vi "lf-condition-1122.vi"() -> ()   [LabVIEW 2019]
panel:
  out "Navigate Tree:Get Parent":string
  out "数字":i32
  in  "sce-pannel":T1 {"pannel"."ID" format="%02x"}
  out "节点列表":T2(array[cluster])
  in  "Action":string(combo) caption="动作"
  in  "节点-操作 9":T3={"ID"=0, "type"="dev", "flag"="", "name"="", "Act"={"Attribute"="dev", "Action"="", "Value"=0.0}} caption="簇 7" {"ID" format="%02x"}
  out "节点引用数组":refnum<vi>[](array[refnum])
  in  "节点-操作 4":T3={"ID"=0, "type"="dev", "flag"="", "name"="", "Act"={"Attribute"="dev", "Action"="", "Value"=0.0}} caption="簇 7" {"ID" format="%02x"}
  in  "节点-操作 3":T3={"ID"=0, "type"="dev", "flag"="", "name"="", "Act"={"Attribute"="dev", "Action"="", "Value"=0.0}} caption="簇 7" {"ID" format="%02x"}
  in  "节点-操作 2":T3={"ID"=0, "type"="dev", "flag"="", "name"="", "Act"={"Attribute"="dev", "Action"="", "Value"=0.0}} caption="簇 7" {"ID" format="%02x"}
  in  "节点-操作":T3={"ID"=0, "type"="dev", "flag"="", "name"="", "Act"={"Attribute"="dev", "Action"="", "Value"=0.0}} caption="簇 7" {"ID" format="%02x"}
  in  "模式列表":T4(array[cluster]) {"sce-pannel-list"."pannel"."ID" format="%02x"}
  in  "节点-操作 5":T3={"ID"=0, "type"="dev", "flag"="", "name"="", "Act"={"Attribute"="dev", "Action"="", "Value"=0.0}} caption="簇 7" {"ID" format="%02x"}
  in  "选项卡控件":enum32{"选项卡 1", "选项卡 2"}(tab)
  in  "面板地址 2":u8 format="%02d"
  in  "添加面板":bool
  in  "单选按钮 2":T5(radio)
  in  "簇 6":T6={"ID"=0, "Attribute"="dev", "Action"="", "name"=""} {"ID" format="%02x"}
  in  "簇 5":T6={"ID"=0, "Attribute"="dev", "Action"="", "name"=""} {"ID" format="%02x"}
  in  "簇 4":T6={"ID"=0, "Attribute"="dev", "Action"="", "name"=""} {"ID" format="%02x"}
  in  "簇 3":T6={"ID"=0, "Attribute"="dev", "Action"="", "name"=""} {"ID" format="%02x"}
  in  "簇 2":T6={"ID"=0, "Attribute"="dev", "Action"="", "name"=""} {"ID" format="%02.0f"}
  in  "簇 1":T6={"ID"=0, "Attribute"="dev", "Action"="", "name"=""} {"ID" format="%02x"}
  in  "节点-操作 26":T3={"ID"=0, "type"="dev", "flag"="", "name"="", "Act"={"Attribute"="dev", "Action"="", "Value"=0.0}} caption="簇 7" {"ID" format="%02x"}
  in  "节点-操作 23":T3={"ID"=0, "type"="dev", "flag"="", "name"="", "Act"={"Attribute"="dev", "Action"="", "Value"=0.0}} caption="簇 7" {"ID" format="%02x"}
  in  "节点-操作 25":T3={"ID"=0, "type"="dev", "flag"="", "name"="", "Act"={"Attribute"="dev", "Action"="", "Value"=0.0}} caption="簇 7" {"ID" format="%02x"}
  in  "节点-操作 24":T3={"ID"=0, "type"="dev", "flag"="", "name"="", "Act"={"Attribute"="dev", "Action"="", "Value"=0.0}} caption="簇 7" {"ID" format="%02x"}
  in  "节点-操作 22":T3={"ID"=0, "type"="dev", "flag"="", "name"="", "Act"={"Attribute"="dev", "Action"="", "Value"=0.0}} caption="簇 7" {"ID" format="%02x"}
  in  "节点-操作 21":T3={"ID"=0, "type"="dev", "flag"="", "name"="", "Act"={"Attribute"="dev", "Action"="", "Value"=0.0}} caption="簇 7" {"ID" format="%02x"}
  in  "面板地址":string(combo)
  in  "模式":string(combo)
  in  "添加设备":bool
  in  "节点-输出":T7(array[cluster])
  in  "场景":string(tree)
  out "node":T7(array[cluster])
  in  "停止":bool
  out "pannel-id-list":string[](array[string])
  out "Node-list":T8(array[cluster])
  in  "Node-model":T9
  in  "pannel-list":T10(array[cluster])
  in  "panel":string(tree)
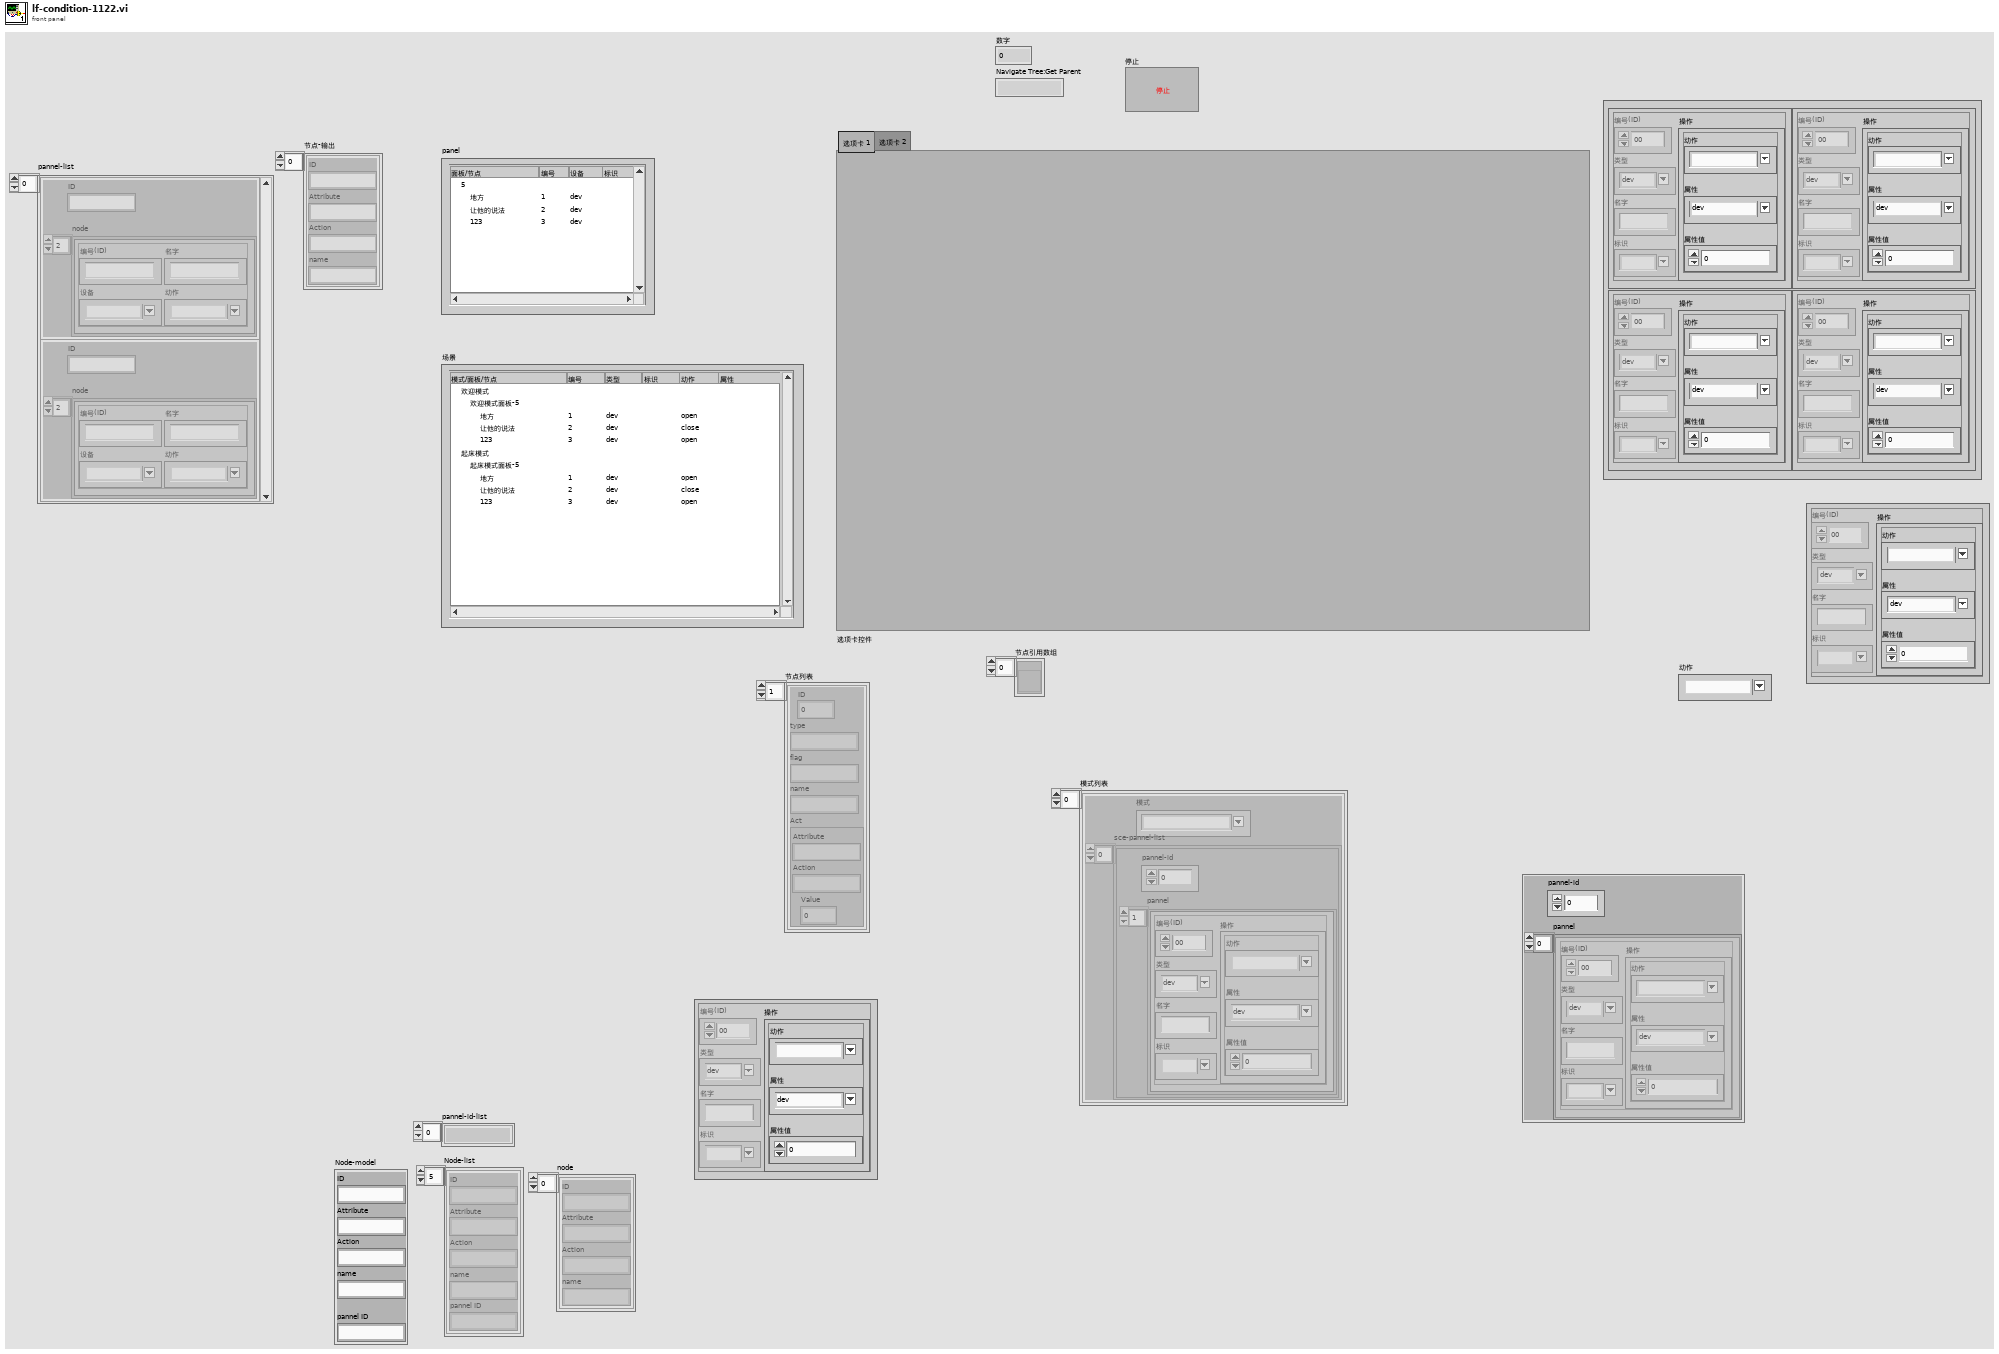
[diagram p1: front panel]
types:
  T1 = cluster{"pannel":cluster{"ID":u8, "type":string, "flag":string, "name":string, "Act":cluster{"Attribute":string, "Action":string, "Value":dbl}}[], "pannel-id":dbl}
  T2 = cluster{"ID":u8, "type":string, "flag":string, "name":string, "Act":cluster{"Attribute":string, "Action":string, "Value":dbl}}[]
  T3 = cluster{"ID":u8, "type":string, "flag":string, "name":string, "Act":cluster{"Attribute":string, "Action":string, "Value":dbl}}
  T4 = cluster{"模式":string, "sce-pannel-list":cluster{"pannel":cluster{"ID":u8, "type":string, "flag":string, "name":string, "Act":cluster{"Attribute":string, "Action":string, "Value":dbl}}[], "pannel-id":dbl}[]}[]
  T5 = enum32{"单键面板", "双键面板", "三键面板", "四键面板", "六键面板", "调光面板"}
  T6 = cluster{"ID":u8, "Attribute":string, "Action":string, "name":string}
  T7 = cluster{"ID":string, "Attribute":string, "Action":string, "name":string}[]
  T8 = cluster{"ID":string, "Attribute":string, "Action":string, "name":string, "pannel ID":string}[]
  T9 = cluster{"ID":string, "Attribute":string, "Action":string, "name":string, "pannel ID":string}
  T10 = cluster{"node":cluster{"ID":string, "Attribute":string, "Action":string, "name":string}[], "ID":string}[]
  T11 = cluster{"node":cluster{"ID":string, "Attribute":string, "Action":string, "name":string}[], "ID":string}
  T12 = enum8{"Enabled", "Disabled", "Disabled and Grayed Out"}
  T13 = cluster{"模式":string, "sce-pannel-list":cluster{"pannel":cluster{"ID":u8, "type":string, "flag":string, "name":string, "Act":cluster{"Attribute":string, "Action":string, "Value":dbl}}[], "pannel-id":dbl}[]}
  T14 = cluster{"ID":u8, "Attribute":string, "Action":string, "name":string}[]
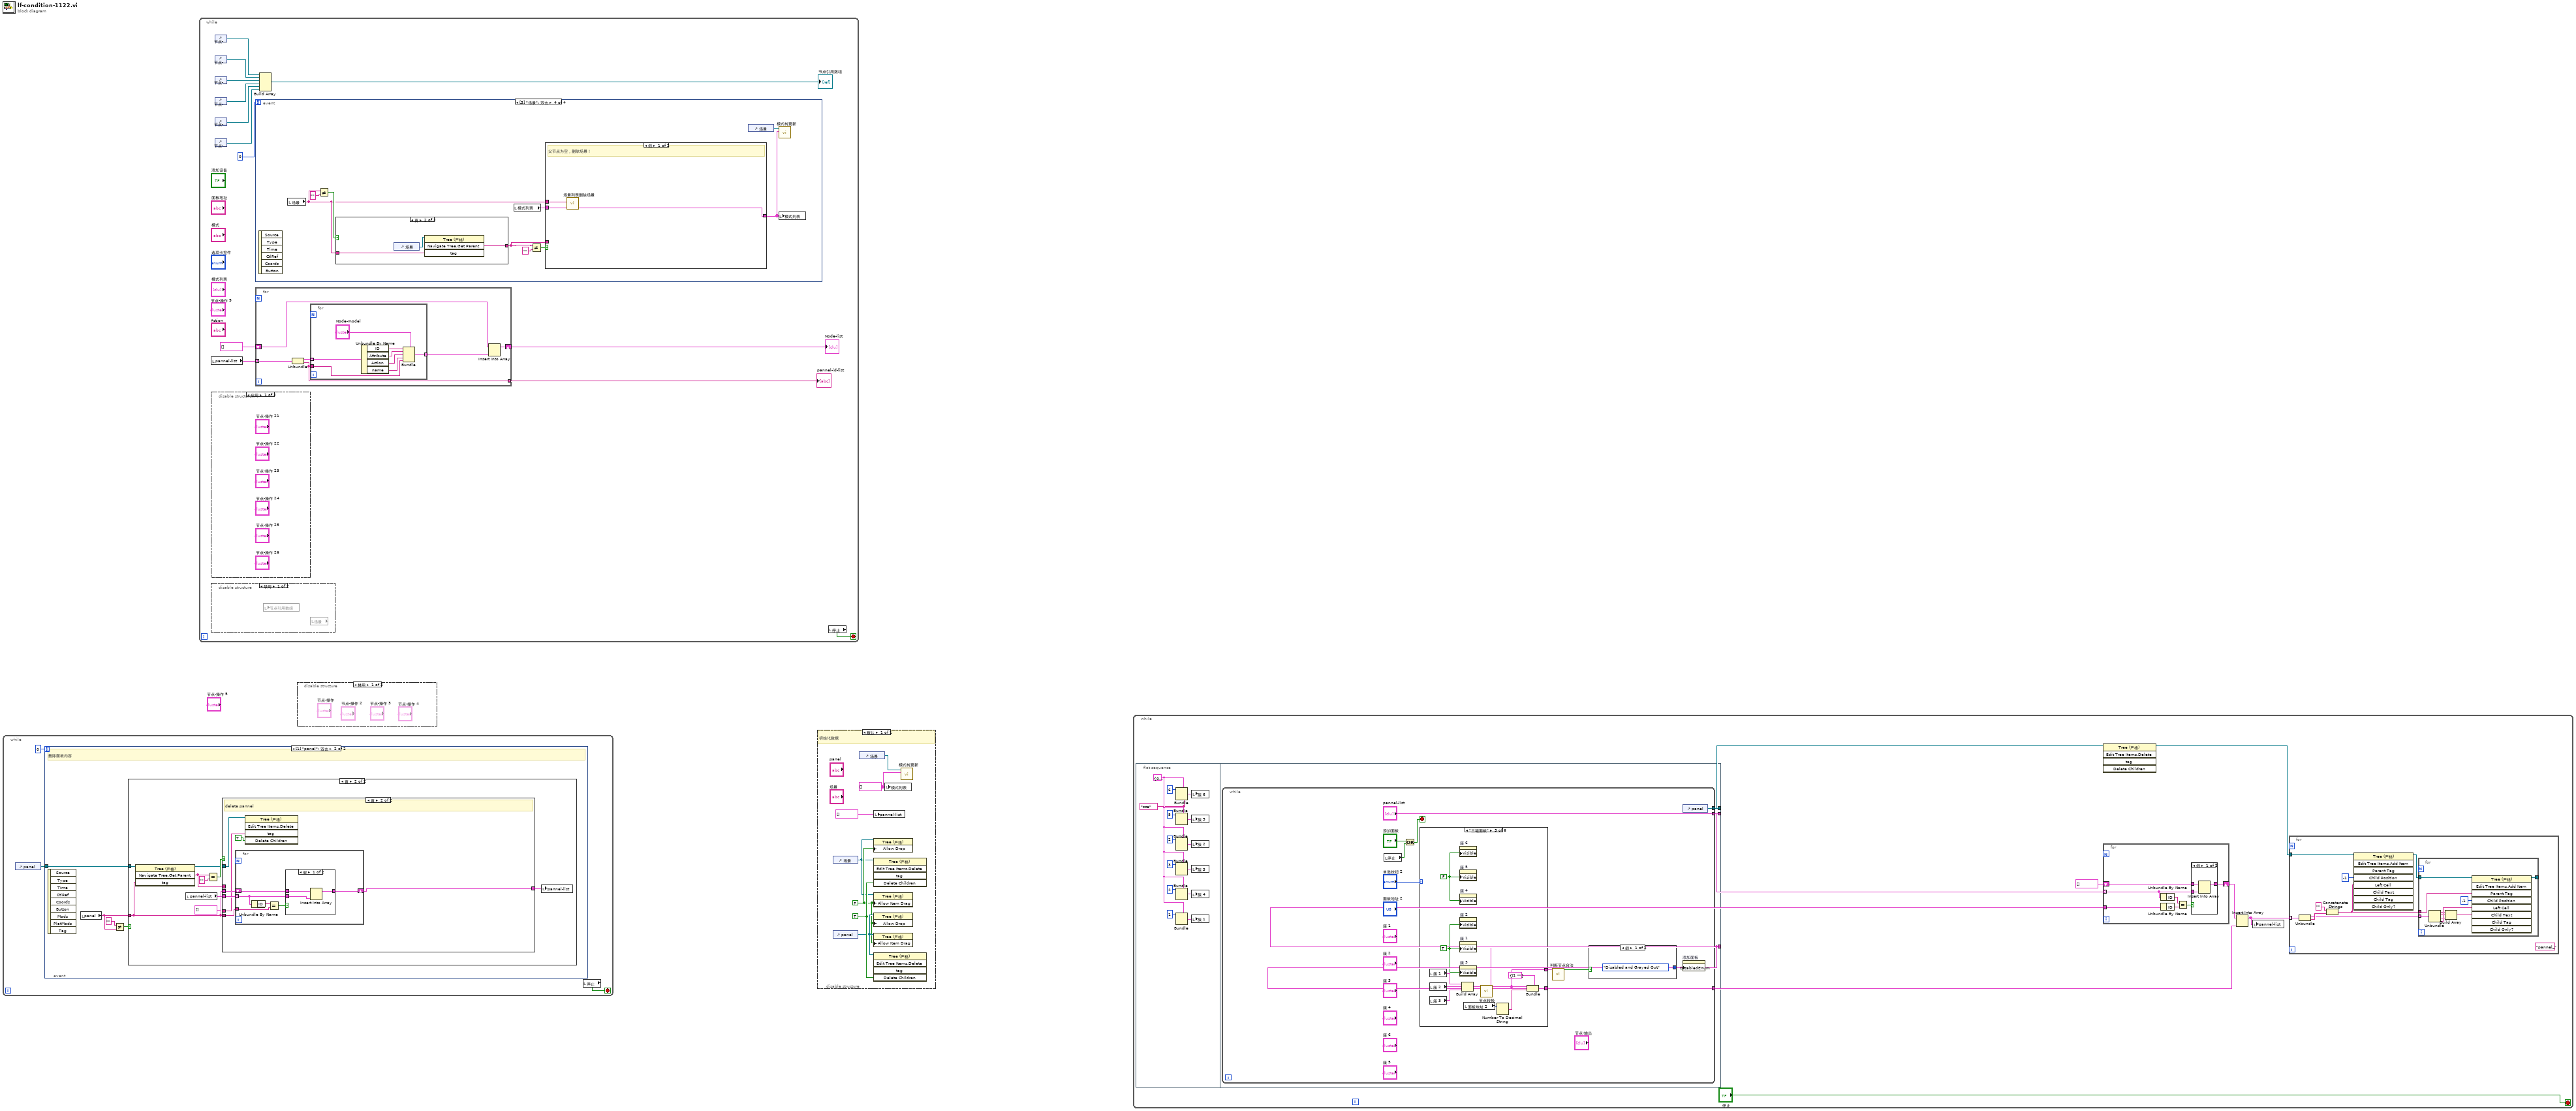
[diagram p0: block diagram]
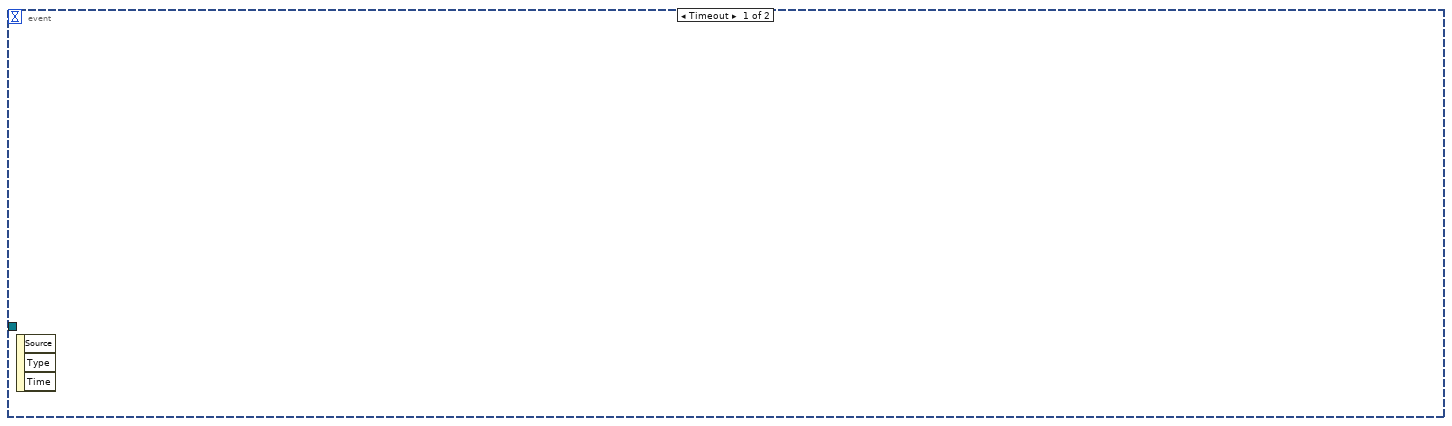
[diagram p3: hidden frame]
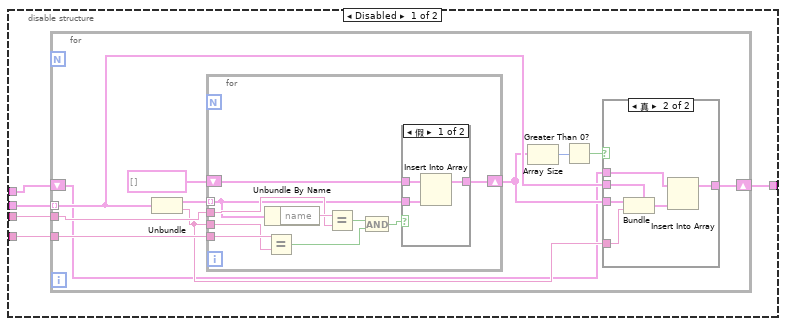
[diagram p6: hidden frame]
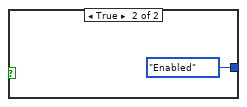
[diagram p10: hidden frame]
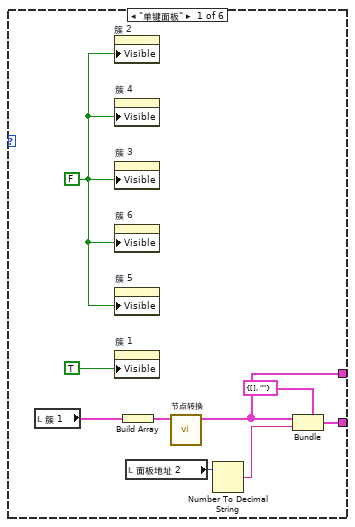
[diagram p11: hidden frame]
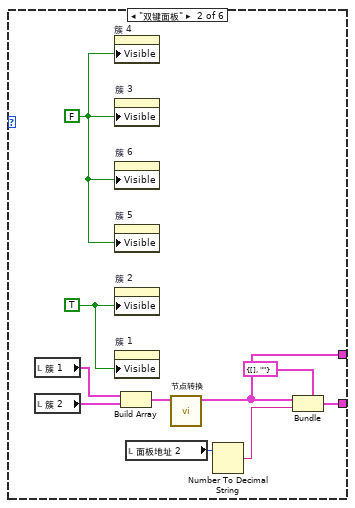
[diagram p12: hidden frame]
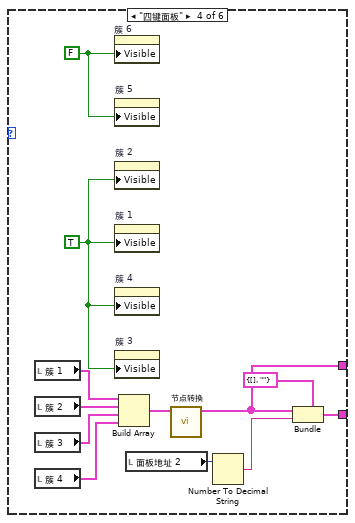
[diagram p13: hidden frame]
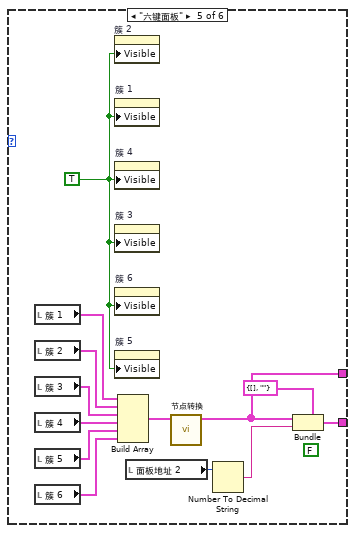
[diagram p14: hidden frame]
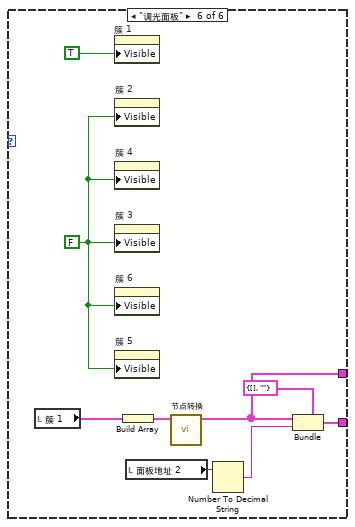
[diagram p15: hidden frame]
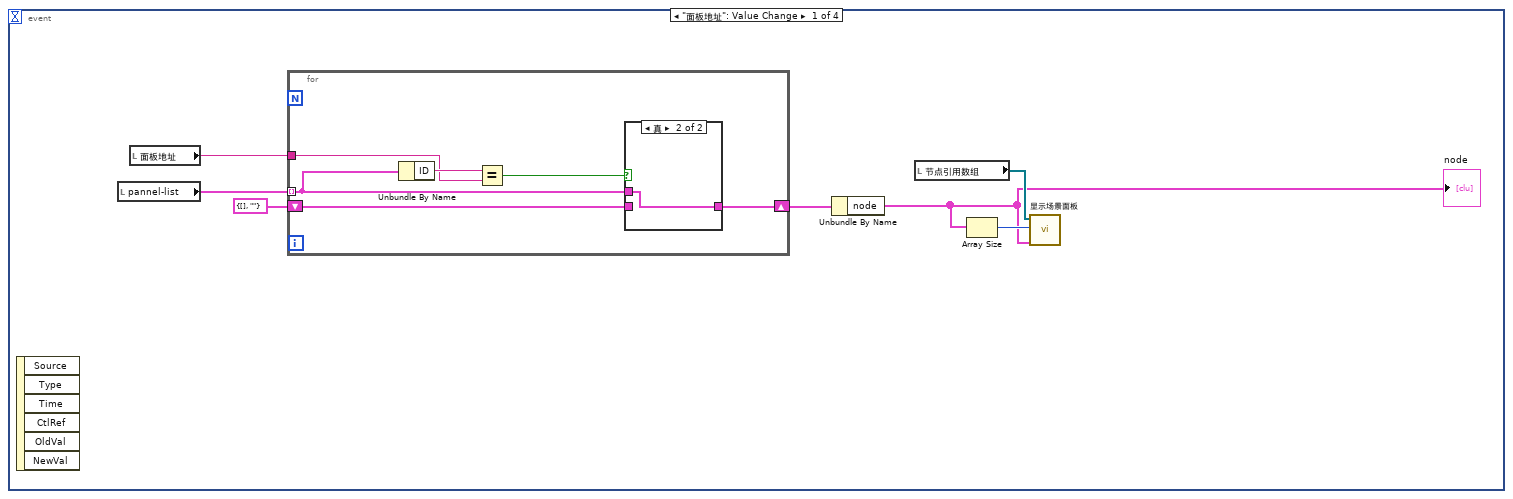
[diagram p19: hidden frame]
diagram:
  n1 = while {
    stop <- w3 stop-if-true
    n2 = control-ref of="panel"() -> (w1:refnum<vi>)
    n3 = event shown="[1] \"panel\": 双击" {
      selector: _ -> [_ _]
      dyn-events: _ -> [_ _]
      timeout: 0 -> [_ _]
      tunnel: w1 -> [_ w7]
      event Timeout {
        n4 = event-data() -> ()  [unwired: 1 in, 3 out]
      }
      event "panel": Double Click {
        # "删除面板内容"
        n5 = event-data() -> ()  [unwired: 1 in, 9 out]
        n6 = local read "panel"() -> (w5:string)
        n7 = Not Equal?(x="", y=w5) -> (x != y?=w6:bool)
        n8 = case shown="真" w6 {
          tunnel: w7 -> [_ w16]
          tunnel: w5 -> [_ w8]
          frame False {
          }
          frame True {
            n9 = invoke class="Tree (严格)" method="Navigate Tree.Get Parent"(reference=w16, "tag"=w8) -> (reference out=w9:refnum<vi>, "Navigate Tree:Get Parent"=w13:string)  [unwired: 2 in, 2 out]
            n10 = local read "pannel-list"() -> (w12:T10)
            n11 = Equal?(x=w13, y="") -> (x = y?=w14:bool)
            n12 = case shown="真" w14 {
              tunnel: w8 -> [w19 w65]
              tunnel: w13 -> [w20 _]
              tunnel: w12 -> [w21 w66]
              tunnel: [w18 w64] -> w11
              tunnel: T10 [] -> [w17 w63]
              tunnel: w9 -> [_ w62]
              tunnel: w8 -> [_ w61]
              frame False {
                # "delete node"
                n13 = disable-structure shown="启用" {
                  disable-tunnel: w21 -> [w26 w59]
                  disable-tunnel: w20 -> [w25 _]
                  disable-tunnel: w19 -> [w24 _]
                  disable-tunnel: [w23 w59] -> w18
                  disable-tunnel: w17 -> [w22 _]
                  frame Disabled {
                    n14 = for {
                      tunnel: w26 -> [w32] mode=indexing
                      tunnel: w25 -> [w36]
                      tunnel: w24 -> [w35]
                      shift-right: [w29] -> w23
                      shift-left: w22 -> [w28]
                      n15 = Unbundle(w32) -> ("node"=w37:T7, "ID"=w30:string)
                      n16 = for {
                        tunnel: w37 -> [w45] mode=indexing
                        tunnel: w30 -> [w53]
                        tunnel: w36 -> [w54]
                        tunnel: w35 -> [w51]
                        shift-right: [w46] -> w31
                        shift-left: T7 [] -> [w47]
                        n17 = Unbundle By Name(w45) -> ("name"=w52:string)
                        n18 = Equal?(x=w54, y=w53) -> (x = y?=w49:bool)
                        n19 = Equal?(x=w52, y=w51) -> (x = y?=w50:bool)
                        n20 = And(x=w50, y=w49) -> (x .and. y?=w48:bool)
                        n21 = case shown="假" w48 {
                          tunnel: w47 -> [w57 w58]
                          tunnel: [w56 w58] -> w46
                          tunnel: w45 -> [w55 _]
                          frame False {
                            n22 = Insert Into Array(array=w57, new element=w55) -> (w56:T7)  [unwired: 1 in]
                          }
                          frame True {
                          }
                        }
                      }
                      n23 = Array Size(array=w31) -> (size(s)=w34:i32)
                      n24 = Greater Than 0?(x=w34) -> (x > 0?=w33:bool)
                      n25 = case shown="真" w33 {
                        tunnel: w32 -> [_ w44]
                        tunnel: w31 -> [_ w43]
                        tunnel: w30 -> [_ w42]
                        tunnel: [w38 w40] -> w29
                        tunnel: w28 -> [w38 w39]
                        frame False {
                        }
                        frame True {
                          n26 = Bundle(cluster=w44, "node"=w43, "ID"=w42) -> (w41:T11)
                          n27 = Insert Into Array(array=w39, new element=w41) -> (w40:T10)  [unwired: 1 in]
                        }
                      }
                    }
                  }
                  frame Enabled {
                  }
                }
              }
              frame True {
                # "delete pannel"
                n28 = for {
                  tunnel: w66 -> [w69] mode=indexing
                  tunnel: w65 -> [w71]
                  shift-right: [w68] -> w64
                  shift-left: w63 -> [w67]
                  n29 = Unbundle By Name(w69) -> ("ID"=w72:string)
                  n30 = Equal?(x=w72, y=w71) -> (x = y?=w70:bool)
                  n31 = case shown="假" w70 {
                    tunnel: w69 -> [w75 _]
                    tunnel: [w74 w76] -> w68
                    tunnel: w67 -> [w73 w76]
                    frame False {
                      n32 = Insert Into Array(array=w73, new element=w75) -> (w74:T10)  [unwired: 1 in]
                    }
                    frame True {
                    }
                  }
                }
                n33 = invoke class="Tree (严格)" method="Edit Tree Items.Delete"(reference=w62, "tag"=w61, "Delete Children"=TRUE ("删除子项？")) -> ()  [unwired: 2 in, 5 out]
              }
            }
            n34 = local write "pannel-list"(w11) -> ()
          }
        }
      }
    }
    n35 = local read "停止"() -> (w3:bool)
  }
  n36 = while {
    stop <- w85 stop-if-true
    n37 = local read "pannel-list"() -> (w86:T10)
    n38 = disable-structure shown="启用" {
      frame Enabled {
      }
      frame Disabled {
      }
    }
    n39 = disable-structure shown="禁用" {
      frame Disabled {
        n40 = local read "节点引用数组"() -> ()  [unwired: 1 in]
        n41 = local read "场景"() -> ()  [unwired: 1 out]
      }
      frame Enabled {
      }
    }
    n42 = control-ref of="节点-操作 21"() -> (w83:refnum<vi>)
    n43 = control-ref of="节点-操作 22"() -> (w82:refnum<vi>)
    n44 = control-ref of="节点-操作 23"() -> (w81:refnum<vi>)
    n45 = control-ref of="节点-操作 24"() -> (w80:refnum<vi>)
    n46 = control-ref of="节点-操作 25"() -> (w79:refnum<vi>)
    n47 = control-ref of="节点-操作 26"() -> (w78:refnum<vi>)
    n48 = event shown="[3] \"场景\": 双击" {
      selector: _ -> [_ _ _ _]
      dyn-events: _ -> [_ _ _ _]
      timeout: 0 -> [_ _ _ _]
      event "面板地址": Value Change {
        n49 = event-data() -> ()  [unwired: 1 in, 6 out]
        n50 = local read "pannel-list"() -> (w93:T10)
        n51 = local read "面板地址"() -> (w94:string)
        n52 = for {
          tunnel: w93 -> [w99] mode=indexing
          tunnel: w94 -> [w101]
          shift-right: [w98] -> w95
          shift-left: T11 {"node"=[], "ID"=""} ("pannel") -> [w97]
          n53 = Unbundle By Name(w99) -> ("ID"=w102:string)
          n54 = Equal?(x=w102, y=w101) -> (x = y?=w100:bool)
          n55 = case shown="真" w100 {
            tunnel: w99 -> [_ w104]
            tunnel: [w103 w104] -> w98
            tunnel: w97 -> [w103 _]
            frame False {
            }
            frame True {
            }
          }
        }
        n56 = Unbundle By Name(w95) -> ("node"=w90:T7)
        "node" <- w90
        n57 = local read "节点引用数组"() -> (w91:refnum<vi>[])
        n58 = Array Size(array=w90) -> (size(s)=w92:i32)
        n59 = call "显示场景面板.vi"("node"=w90, "数目"=w92, "节点引用数组"=w91) -> ()  [unwired: 9 in]
      }
      event Timeout {
        n60 = event-data() -> ()  [unwired: 1 in, 3 out]
        n61 = local read "pannel-id-list"() -> (w105:string[])
        n62 = local read "节点引用数组"() -> (w107:refnum<vi>[])
        n63 = property on="面板地址" class="CmbBox"("Strings[]"=w105) -> ()  [unwired: 2 in, 2 out]
        n64 = call "获取合法面板.vi"("节点引用数组"=w107) -> ("合法"=w106:bool)  [unwired: 9 in, 1 out]
        n65 = case shown="真" w106 {
          frame False {
            n66 = property on="添加设备" class="Bool (严格)"("DisabledEnum"=T12."Disabled and Grayed Out" ("禁用")) -> ()  [unwired: 2 in, 2 out]
          }
          frame True {
            n67 = property on="添加设备" class="Bool (严格)"("DisabledEnum"=T12."Enabled" ("禁用")) -> ()  [unwired: 2 in, 2 out]
          }
        }
      }
      event "添加设备": Value Change {
        n68 = event-data() -> ()  [unwired: 1 in, 6 out]
        n69 = local write "添加设备"(FALSE ("添加设备")) -> ()
        n70 = local read "模式列表"() -> (w119:T4)
        n71 = local read "模式"() -> (w116:string)
        n72 = local read "节点引用数组"() -> (w124:refnum<vi>[])
        n73 = for {
          tunnel: w119 -> [w129] mode=indexing
          tunnel: w116 -> [w132]
          shift-right: [w130] -> w117
          shift-left: T13 {"模式"="", "sce-pannel-list"=[]} ("模式 2") -> [w128]
          shift-right: [w127] -> w114
          shift-left: T4 [] -> [w126]
          n74 = Unbundle By Name(w129) -> ("模式"=w133:string)
          n75 = Equal?(x=w133, y=w132) -> (x = y?=w131:bool)
          n76 = case shown="真" w131 {
            tunnel: [w137 w139] -> w130
            tunnel: w129 -> [w136 w139]
            tunnel: w128 -> [w137 _]
            tunnel: [w135 w138] -> w127
            tunnel: w126 -> [w134 w138]
            frame False {
              n77 = Insert Into Array(array=w134, new element=w136) -> (w135:T4)  [unwired: 1 in]
            }
            frame True {
            }
          }
        }
        n78 = call "获取合法节点列表.vi"("节点引用数组"=w124) -> ("节点列表"=w122:T2)  [unwired: 10 in]
        "节点列表" <- w122
        n79 = local read "面板地址"() -> (w123:string)
        n80 = Decimal String To Number(string=w123) -> (number=w121:i32)  [unwired: 2 in, 1 out]
        n81 = Bundle(cluster=T1 {"pannel"=[], "pannel-id"=0.0} ("sce-pannel"), "pannel"=w122, "pannel-id"=w121) -> (w115:T1)
        n82 = call "模式插入面板.vi"("模式面板"=w115, "模式选择"=w116, "模式 input"=w117) -> ("模式 output"=w113:T13)  [unwired: 8 in]
        n83 = control-ref of="场景"() -> (w111:refnum<vi>)
        n84 = Insert Into Array(array=w114, new element=w113) -> (w112:T4)  [unwired: 1 in]
        n85 = call "模式树更新.vi"("模式列表-new"=w112, "模式树形引用"=w111) -> ()  [unwired: 8 in, 2 out]
        n86 = local write "模式列表"(w112) -> ()
      }
      event "场景": Double Click {
        n87 = event-data() -> ()  [unwired: 1 in, 6 out]
        n88 = local read "场景"() -> (w143:string)
        n89 = Not Equal?(x=w143, y="") -> (x != y?=w148:bool)
        n90 = case shown="真" w148 {
          tunnel: w143 -> [_ w169]
          tunnel: ["" ("y") w168] -> w142
          frame False {
          }
          frame True {
            n91 = control-ref of="场景"() -> (w170:refnum<vi>)
            n92 = invoke class="Tree (严格)" method="Navigate Tree.Get Parent"(reference=w170, "tag"=w169) -> ("Navigate Tree:Get Parent"=w168:string)  [unwired: 2 in, 3 out]
          }
        }
        n93 = local read "模式列表"() -> (w144:T4)
        n94 = Not Equal?(x=w142, y="") -> (x != y?=w145:bool)
        n95 = case shown="假" w145 {
          tunnel: w143 -> [w151 w158]
          tunnel: w144 -> [w150 w154]
          tunnel: [w149 w153] -> w141
          tunnel: w142 -> [_ w152]
          frame False {
            # "父节点为空，删除场景！"
            n96 = call "场景列表删除场景.vi"("模式列表 new"=w150, "场景"=w151) -> ("模式列表 new output"=w149:T4)  [unwired: 8 in, 1 out]
          }
          frame True {
            # "父节点不为空"
            n97 = Match Pattern(string=w158, regular expression="-[0-9]+" ("正则表达式")) -> (match substring=w156:string)  [unwired: 1 in, 3 out]
            n98 = Not Equal?(x=w156, y="") -> (x != y?=w155:bool)
            n99 = case shown="真" w155 {
              tunnel: w156 -> [_ w166]
              tunnel: w154 -> [w160 w164]
              tunnel: [w160 w163] -> w153
              tunnel: w152 -> [_ w161]
              frame False {
              }
              frame True {
                n100 = Decimal String To Number(string=w166) -> (number=w165:i32)  [unwired: 2 in, 1 out]
                "数字" <- w165
                n101 = Absolute Value(x=w165) -> (abs(x)=w162:i32)
                n102 = call "模式列表删除面板.vi"("pannel ID"=w162, "模式"=w161, "模式列表"=w164) -> ("模式列表 output"=w163:T4)  [unwired: 8 in]
              }
            }
            "Navigate Tree:Get Parent" <- w152
          }
        }
        n103 = control-ref of="场景"() -> (w140:refnum<vi>)
        n104 = call "模式树更新.vi"("模式列表-new"=w141, "模式树形引用"=w140) -> ()  [unwired: 8 in, 2 out]
        n105 = local write "模式列表"(w141) -> ()
      }
    }
    n106 = for {
      tunnel: w86 -> [w176] mode=indexing
      shift-right: [w171] -> w89
      shift-left: T8 [] -> [w173]
      tunnel: [w174] -> w87 mode=indexing
      n107 = Unbundle(w176) -> ("node"=w175:T7, "ID"=w174:string)
      n108 = for {
        tunnel: w175 -> [w184] mode=indexing
        tunnel: w174 -> [w178]
        tunnel: [w177] -> w172 mode=indexing
        n109 = Unbundle By Name(w184) -> ("ID"=w182:string, "Attribute"=w181:string, "Action"=w179:string, "name"=w180:string)
        n110 = Bundle(cluster="Node-model", "ID"=w182, "Attribute"=w181, "Action"=w179, "name"=w180, "pannel ID"=w178) -> (w177:T9)
      }
      n111 = Insert Into Array(array=w173, new element=w172) -> (w171:T8)  [unwired: 1 in]
    }
    "Node-list" <- w89
    "pannel-id-list" <- w87
    n112 = Build Array(w83, w82, w81, w80, w79, w78) -> (→"节点引用数组":refnum<vi>[])
    n113 = local read "停止"() -> (w85:bool)
  }
  n114 = disable-structure shown="禁用" {
    frame Disabled {
    }
    frame Enabled {
    }
  }
  n115 = disable-structure shown="默认" {
    frame Enabled {
      w185 = T4 [] ("模式列表")
      w191 = TRUE ("删除子项？")
      w188 = FALSE ("拖曳/放置:允许放置")
      # "初始化数据"
      n116 = control-ref of="场景"() -> (w187:refnum<vi>)
      n117 = control-ref of="panel"() -> (w189:refnum<vi>)
      n118 = control-ref of="场景"() -> (w186:refnum<vi>)
      n119 = local write "pannel-list"(T10 [] ("pannel-list")) -> ()
      n120 = property class="Tree (严格)"(reference=w187, "Allow Drop"=w188) -> ()  [unwired: 1 in, 2 out]
      n121 = invoke class="Tree (严格)" method="Edit Tree Items.Delete"(reference=w187, "Delete Children"=w191) -> ()  [unwired: 3 in, 5 out]
      n122 = property class="Tree (严格)"(reference=w187, "Allow Item Drag"=w188) -> ()  [unwired: 1 in, 2 out]
      n123 = property class="Tree (严格)"(reference=w189, "Allow Drop"=w188) -> ()  [unwired: 1 in, 2 out]
      n124 = property class="Tree (严格)"(reference=w189, "Allow Item Drag"=w188) -> ()  [unwired: 1 in, 2 out]
      n125 = invoke class="Tree (严格)" method="Edit Tree Items.Delete"(reference=w189, "Delete Children"=w191) -> ()  [unwired: 3 in, 5 out]
      n126 = local write "模式列表"(w185) -> ()
      n127 = call "模式树更新.vi"("模式列表-new"=w185, "模式树形引用"=w186) -> ()  [unwired: 8 in, 2 out]
    }
  }
  n128 = while {
    stop <- "停止" stop-if-true
    n129 = flat-sequence {
      tunnel: [w216] -> w194
      tunnel: [w215] -> w193
      tunnel: [w214] -> w192
      frame #0 {
        w202 = "sce" ("Attribute")
        w207 = T6 {"ID"=0, "Attribute"="dev", "Action"="", "name"=""} ("簇 1")
        n130 = Bundle(cluster=w207, "ID"=u8 6, "Attribute"=w202) -> (w209:T6)  [unwired: 2 in]
        n131 = Bundle(cluster=w207, "ID"=u8 5, "Attribute"=w202) -> (w210:T6)  [unwired: 2 in]
        n132 = Bundle(cluster=w207, "ID"=u8 2) -> (w211:T6)  [unwired: 3 in]
        n133 = Bundle(cluster=w207, "ID"=u8 3) -> (w212:T6)  [unwired: 3 in]
        n134 = Bundle(cluster=w207, "ID"=u8 4) -> (w213:T6)  [unwired: 3 in]
        n135 = Bundle(cluster=w207, "ID"=u8 1) -> (w208:T6)  [unwired: 3 in]
        n136 = local write "簇 6"(w209) -> ()
        n137 = local write "簇 5"(w210) -> ()
        n138 = local write "簇 2"(w211) -> ()
        n139 = local write "簇 3"(w212) -> ()
        n140 = local write "簇 4"(w213) -> ()
        n141 = local write "簇 1"(w208) -> ()
      }
      frame #1 {
        n142 = while {
          tunnel: [w223] -> w216
          tunnel: [w221] -> w215
          tunnel: ["pannel-list"] -> w214
          stop <- w224 stop-if-true
          n143 = local read "停止"() -> (w222:bool)
          n144 = Or(x="添加面板", y=w222) -> (x .or. y?=w224:bool)
          n145 = case shown="\"三键面板\"" "单选按钮 2" {
            tunnel: [w234 w244 w249 w263 w275 w288] -> w223
            tunnel: [w229 w238 w248 w261 w271 w284] -> w219
            frame "单键面板" {
              w236 = FALSE
              n146 = local read "簇 1"() -> (w231:T6)
              n147 = property on="簇 2" class="Clust (严格)"("Visible"=w236) -> ()  [unwired: 2 in, 2 out]
              n148 = property on="簇 4" class="Clust (严格)"("Visible"=w236) -> ()  [unwired: 2 in, 2 out]
              n149 = property on="簇 3" class="Clust (严格)"("Visible"=w236) -> ()  [unwired: 2 in, 2 out]
              n150 = property on="簇 6" class="Clust (严格)"("Visible"=w236) -> ()  [unwired: 2 in, 2 out]
              n151 = property on="簇 5" class="Clust (严格)"("Visible"=w236) -> ()  [unwired: 2 in, 2 out]
              n152 = property on="簇 1" class="Clust (严格)"("Visible"=TRUE) -> ()  [unwired: 2 in, 2 out]
              n153 = Build Array(w231) -> (w230:T14)
              n154 = local read "面板地址 2"() -> (w233:u8)
              n155 = call "节点转换.vi"("节点"=w230) -> ("节点-输出"=w229:T7)  [unwired: 10 in]
              n156 = Number To Decimal String(number=w233) -> (decimal integer string=w232:string)  [unwired: 1 in]
              n157 = Bundle(cluster=T11 {"node"=[], "ID"=""} ("pannel"), "node"=w229, "ID"=w232) -> (w234:T11)
            }
            frame "双键面板" {
              w247 = FALSE
              w246 = TRUE
              n158 = local read "簇 1"() -> (w241:T6)
              n159 = local read "簇 2"() -> (w240:T6)
              n160 = property on="簇 4" class="Clust (严格)"("Visible"=w247) -> ()  [unwired: 2 in, 2 out]
              n161 = property on="簇 3" class="Clust (严格)"("Visible"=w247) -> ()  [unwired: 2 in, 2 out]
              n162 = property on="簇 6" class="Clust (严格)"("Visible"=w247) -> ()  [unwired: 2 in, 2 out]
              n163 = property on="簇 5" class="Clust (严格)"("Visible"=w247) -> ()  [unwired: 2 in, 2 out]
              n164 = property on="簇 2" class="Clust (严格)"("Visible"=w246) -> ()  [unwired: 2 in, 2 out]
              n165 = property on="簇 1" class="Clust (严格)"("Visible"=w246) -> ()  [unwired: 2 in, 2 out]
              n166 = Build Array(w241, w240) -> (w239:T14)
              n167 = local read "面板地址 2"() -> (w243:u8)
              n168 = call "节点转换.vi"("节点"=w239) -> ("节点-输出"=w238:T7)  [unwired: 10 in]
              n169 = Number To Decimal String(number=w243) -> (decimal integer string=w242:string)  [unwired: 1 in]
              n170 = Bundle(cluster=T11 {"node"=[], "ID"=""} ("pannel"), "node"=w238, "ID"=w242) -> (w244:T11)
            }
            frame "三键面板" {
              w258 = FALSE
              w257 = TRUE
              n171 = local read "簇 1"() -> (w256:T6)
              n172 = local read "簇 2"() -> (w255:T6)
              n173 = local read "簇 3"() -> (w254:T6)
              n174 = property on="簇 6" class="Clust (严格)"("Visible"=w258) -> ()  [unwired: 2 in, 2 out]
              n175 = property on="簇 5" class="Clust (严格)"("Visible"=w258) -> ()  [unwired: 2 in, 2 out]
              n176 = property on="簇 4" class="Clust (严格)"("Visible"=w258) -> ()  [unwired: 2 in, 2 out]
              n177 = property on="簇 2" class="Clust (严格)"("Visible"=w257) -> ()  [unwired: 2 in, 2 out]
              n178 = property on="簇 1" class="Clust (严格)"("Visible"=w257) -> ()  [unwired: 2 in, 2 out]
              n179 = property on="簇 3" class="Clust (严格)"("Visible"=w257) -> ()  [unwired: 2 in, 2 out]
              n180 = Build Array(w256, w255, w254) -> (w252:T14)
              n181 = local read "面板地址 2"() -> (w251:u8)
              n182 = call "节点转换.vi"("节点"=w252) -> ("节点-输出"=w248:T7)  [unwired: 10 in]
              n183 = Number To Decimal String(number=w251) -> (decimal integer string=w250:string)  [unwired: 1 in]
              n184 = Bundle(cluster=T11 {"node"=[], "ID"=""} ("pannel"), "node"=w248, "ID"=w250) -> (w249:T11)
            }
            frame "四键面板" {
              w270 = FALSE
              w269 = TRUE
              n185 = local read "簇 1"() -> (w266:T6)
              n186 = local read "簇 2"() -> (w265:T6)
              n187 = local read "簇 3"() -> (w267:T6)
              n188 = local read "簇 4"() -> (w268:T6)
              n189 = property on="簇 6" class="Clust (严格)"("Visible"=w270) -> ()  [unwired: 2 in, 2 out]
              n190 = property on="簇 5" class="Clust (严格)"("Visible"=w270) -> ()  [unwired: 2 in, 2 out]
              n191 = property on="簇 2" class="Clust (严格)"("Visible"=w269) -> ()  [unwired: 2 in, 2 out]
              n192 = property on="簇 1" class="Clust (严格)"("Visible"=w269) -> ()  [unwired: 2 in, 2 out]
              n193 = property on="簇 4" class="Clust (严格)"("Visible"=w269) -> ()  [unwired: 2 in, 2 out]
              n194 = property on="簇 3" class="Clust (严格)"("Visible"=w269) -> ()  [unwired: 2 in, 2 out]
              n195 = Build Array(w266, w265, w267, w268) -> (w262:T14)
              n196 = local read "面板地址 2"() -> (w260:u8)
              n197 = call "节点转换.vi"("节点"=w262) -> ("节点-输出"=w261:T7)  [unwired: 10 in]
              n198 = Number To Decimal String(number=w260) -> (decimal integer string=w259:string)  [unwired: 1 in]
              n199 = Bundle(cluster=T11 {"node"=[], "ID"=""} ("pannel"), "node"=w261, "ID"=w259) -> (w263:T11)
            }
            frame "六键面板" {
              (unwired) FALSE
              w283 = TRUE
              n200 = local read "簇 1"() -> (w278:T6)
              n201 = local read "簇 2"() -> (w277:T6)
              n202 = local read "簇 3"() -> (w279:T6)
              n203 = local read "簇 4"() -> (w280:T6)
              n204 = local read "簇 5"() -> (w281:T6)
              n205 = local read "簇 6"() -> (w282:T6)
              n206 = property on="簇 2" class="Clust (严格)"("Visible"=w283) -> ()  [unwired: 2 in, 2 out]
              n207 = property on="簇 1" class="Clust (严格)"("Visible"=w283) -> ()  [unwired: 2 in, 2 out]
              n208 = property on="簇 4" class="Clust (严格)"("Visible"=w283) -> ()  [unwired: 2 in, 2 out]
              n209 = property on="簇 3" class="Clust (严格)"("Visible"=w283) -> ()  [unwired: 2 in, 2 out]
              n210 = property on="簇 6" class="Clust (严格)"("Visible"=w283) -> ()  [unwired: 2 in, 2 out]
              n211 = property on="簇 5" class="Clust (严格)"("Visible"=w283) -> ()  [unwired: 2 in, 2 out]
              n212 = Build Array(w278, w277, w279, w280, w281, w282) -> (w272:T14)
              n213 = local read "面板地址 2"() -> (w274:u8)
              n214 = call "节点转换.vi"("节点"=w272) -> ("节点-输出"=w271:T7)  [unwired: 10 in]
              n215 = Number To Decimal String(number=w274) -> (decimal integer string=w273:string)  [unwired: 1 in]
              n216 = Bundle(cluster=T11 {"node"=[], "ID"=""} ("pannel"), "node"=w271, "ID"=w273) -> (w275:T11)
            }
            frame "调光面板" {
              w292 = FALSE
              n217 = local read "簇 1"() -> (w290:T6)
              n218 = property on="簇 1" class="Clust (严格)"("Visible"=TRUE) -> ()  [unwired: 2 in, 2 out]
              n219 = property on="簇 2" class="Clust (严格)"("Visible"=w292) -> ()  [unwired: 2 in, 2 out]
              n220 = property on="簇 4" class="Clust (严格)"("Visible"=w292) -> ()  [unwired: 2 in, 2 out]
              n221 = property on="簇 3" class="Clust (严格)"("Visible"=w292) -> ()  [unwired: 2 in, 2 out]
              n222 = property on="簇 6" class="Clust (严格)"("Visible"=w292) -> ()  [unwired: 2 in, 2 out]
              n223 = property on="簇 5" class="Clust (严格)"("Visible"=w292) -> ()  [unwired: 2 in, 2 out]
              n224 = Build Array(w290) -> (w285:T14)
              n225 = local read "面板地址 2"() -> (w287:u8)
              n226 = call "节点转换.vi"("节点"=w285) -> ("节点-输出"=w284:T7)  [unwired: 10 in]
              n227 = Number To Decimal String(number=w287) -> (decimal integer string=w286:string)  [unwired: 1 in]
              n228 = Bundle(cluster=T11 {"node"=[], "ID"=""} ("pannel"), "node"=w284, "ID"=w286) -> (w288:T11)
            }
          }
          n229 = call "判断节点合法.vi"("节点数组"=w219) -> ("合法"=w217:bool)  [unwired: 10 in]
          n230 = case shown="假" w217 {
            tunnel: [T12."Disabled and Grayed Out" ("禁用") T12."Enabled" ("禁用")] -> w218
            frame False {
            }
            frame True {
            }
          }
          n231 = control-ref of="panel"() -> (w221:refnum<vi>)
          n232 = property on="添加面板" class="Bool"("DisabledEnum"=w218) -> ()  [unwired: 2 in, 2 out]
        }
      }
    }
    n233 = invoke class="Tree (严格)" method="Edit Tree Items.Delete"(reference=w193) -> (reference out=w198:refnum<vi>)  [unwired: 4 in, 4 out]
    n234 = for {
      tunnel: w194 -> [w294]
      tunnel: w192 -> [w293] mode=indexing
      shift-right: [w295] -> w197
      shift-left: T10 [] -> [w296]
      n235 = Unbundle By Name(w293) -> ("ID"=w299:string)
      n236 = Unbundle By Name(w294) -> ("ID"=w298:string)
      n237 = Equal?(x=w299, y=w298) -> (x = y?=w297:bool)
      n238 = case shown="假" w297 {
        tunnel: w296 -> [w302 w303]
        tunnel: [w301 w303] -> w295
        tunnel: w293 -> [w300 _]
        frame False {
          n239 = Insert Into Array(array=w302, new element=w300) -> (w301:T10)  [unwired: 1 in]
        }
        frame True {
        }
      }
    }
    n240 = Insert Into Array(array=w197, new element=w194) -> (w196:T10)  [unwired: 1 in]
    n241 = local write "pannel-list"(w196) -> ()
    n242 = for {
      tunnel: w196 -> [w311] mode=indexing
      tunnel: w198 -> [w305]
      (unwired) "pannel_" ("字符串")
      n243 = Unbundle(w311) -> ("node"=w308:T7, "ID"=w310:string)
      n244 = Concatenate Strings("" ("字符串"), w310) -> (w307:string)
      n245 = invoke class="Tree (严格)" method="Edit Tree Items.Add Item"(reference=w305, "Child Position"=-1 ("子项位置"), "Left Cell"=w307) -> (reference out=w306:refnum<vi>)  [unwired: 6 in, 8 out]
      n246 = for {
        tunnel: w308 -> [w319] mode=indexing
        tunnel: w306 -> [w321]
        tunnel: w307 -> [w320]
        tunnel: [w317] -> _
        n247 = Unbundle(w319) -> ("ID"=w316:string, "Attribute"=w315:string, "Action"=w314:string, "name"=w318:string)
        n248 = Build Array(w316, w315, w314) -> (w313:string[])
        n249 = invoke class="Tree (严格)" method="Edit Tree Items.Add Item"(reference=w321, "Parent Tag"=w320, "Child Position"=-1 ("子项位置"), "Left Cell"=w318, "Child Text"=w313) -> (reference out=w317:refnum<vi>)  [unwired: 4 in, 8 out]
      }
    }
  }
